vi "qrpostionM.vi"() -> ()   [LabVIEW 2019]
uses:
  <vilib>/vision/Instrument.llb/QR Code Report.ctl
  <vilib>/vision/Instrument.llb/QR Code Model Type.ctl
  <vilib>/vision/Instrument.llb/QR Code Stream Mode Type.ctl
  <vilib>/vision/Instrument.llb/Data Matrix Polarity.ctl
  <vilib>/vision/Instrument.llb/Demodulation Mode.ctl
  <vilib>/vision/Instrument.llb/Cell Sample Size.ctl
  <vilib>/vision/Instrument.llb/Cell Filter Mode.ctl
panel:
  out "Image Out 2":T1(plugin-control)
  in  "Stop (F)":bool
  out "Image Out":T1(plugin-control)
  out "Lx":dbl
  out "Rx":dbl
  out "Ly":i32
  out "Ry":i32
  out "QR Barcode Report (2D Barcode Reader 1)":T2={"Found?"=FALSE, "Data"="", "Bounding Box"=[], "Errors Corrected"=0, "Dimensions (Rows/Cols)"=0, "Version"=0, "QR Model"=3, "Stream Mode"=0, "Barcode Polarity"=-2, "Mirrored?"=FALSE, "Append Stream Position"=0, "Size of Append Stream"=0, "First EAN-128 ID"=0, "First Alternate Language ID"=0, "Append Stream ID"=0, "Minimum Edge Strength"=30, "Demodulation Mode"=-2, "Cell Sample Size"=-2, "Cell Filter Mode"=-2} {"Append Stream ID" format="%x"; "Cell Filter Mode" items=["Auto-detect"=-2, "Average"=0, "Median"=1, "Central Average"=2, "High Average"=3, "Low Average"=4, "Very High Average"=5, "Very Low Average"=6, "All Filters"=8]; "Cell Sample Size" items=["Auto-detect"=-2, "1x1"=1, "2x2"=2, "3x3"=3, "4x4"=4, "5x5"=5, "6x6"=6, "7x7"=7]; "Demodulation Mode" items=["Auto-detect"=-2, "Histogram"=0, "Local Contrast"=1, "Combination"=2, "All"=3]; "Barcode Polarity" items=["Auto-detect"=-2, "Black on White"=0, "White on Black"=1]; "Stream Mode" items=["Auto-detect", "Numeric", "AlphaNumeric", "Mixed", "Raw Bytes", "UCC/EAN-128 - In Tokens", "UCC/EAN-128 - In Data", "Extended Character Interpretation", "Kanji"]; "QR Model" items=["Auto Detect", "Micro", "Model 1", "Model 2"]; "Version" max=40 step=1}
  out "Data":string
  out "Array":string[][](array[string])
  out "Particle Measurements (Pixels) (Particle Analysis 1)":dbl[][](array[numeric]) format="%.2f"
  out "subarray":dbl[](array[numeric])
  out "min Y":dbl
  out "min X":dbl
  out "R1":string[](array[string])
  out "R2":string[](array[string])
  out "R3":string[](array[string])
  out "R4":string[](array[string])
  out "R5":string[](array[string])
  out "R11":string
  out "R12":string
  out "R21":string
  out "R22":string
  out "R31":string
  out "R32":string
  out "R41":string
  out "R42":string
  out "R51":string
  out "R52":string
  out "R13":string
  out "R14":string
  out "R15":string
  out "R23":string
  out "R24":string
  out "R25":string
  out "R33":string
  out "R34":string
  out "R35":string
  out "R43":string
  out "R44":string
  out "R45":string
  out "R53":string
  out "R54":string
  out "R55":string
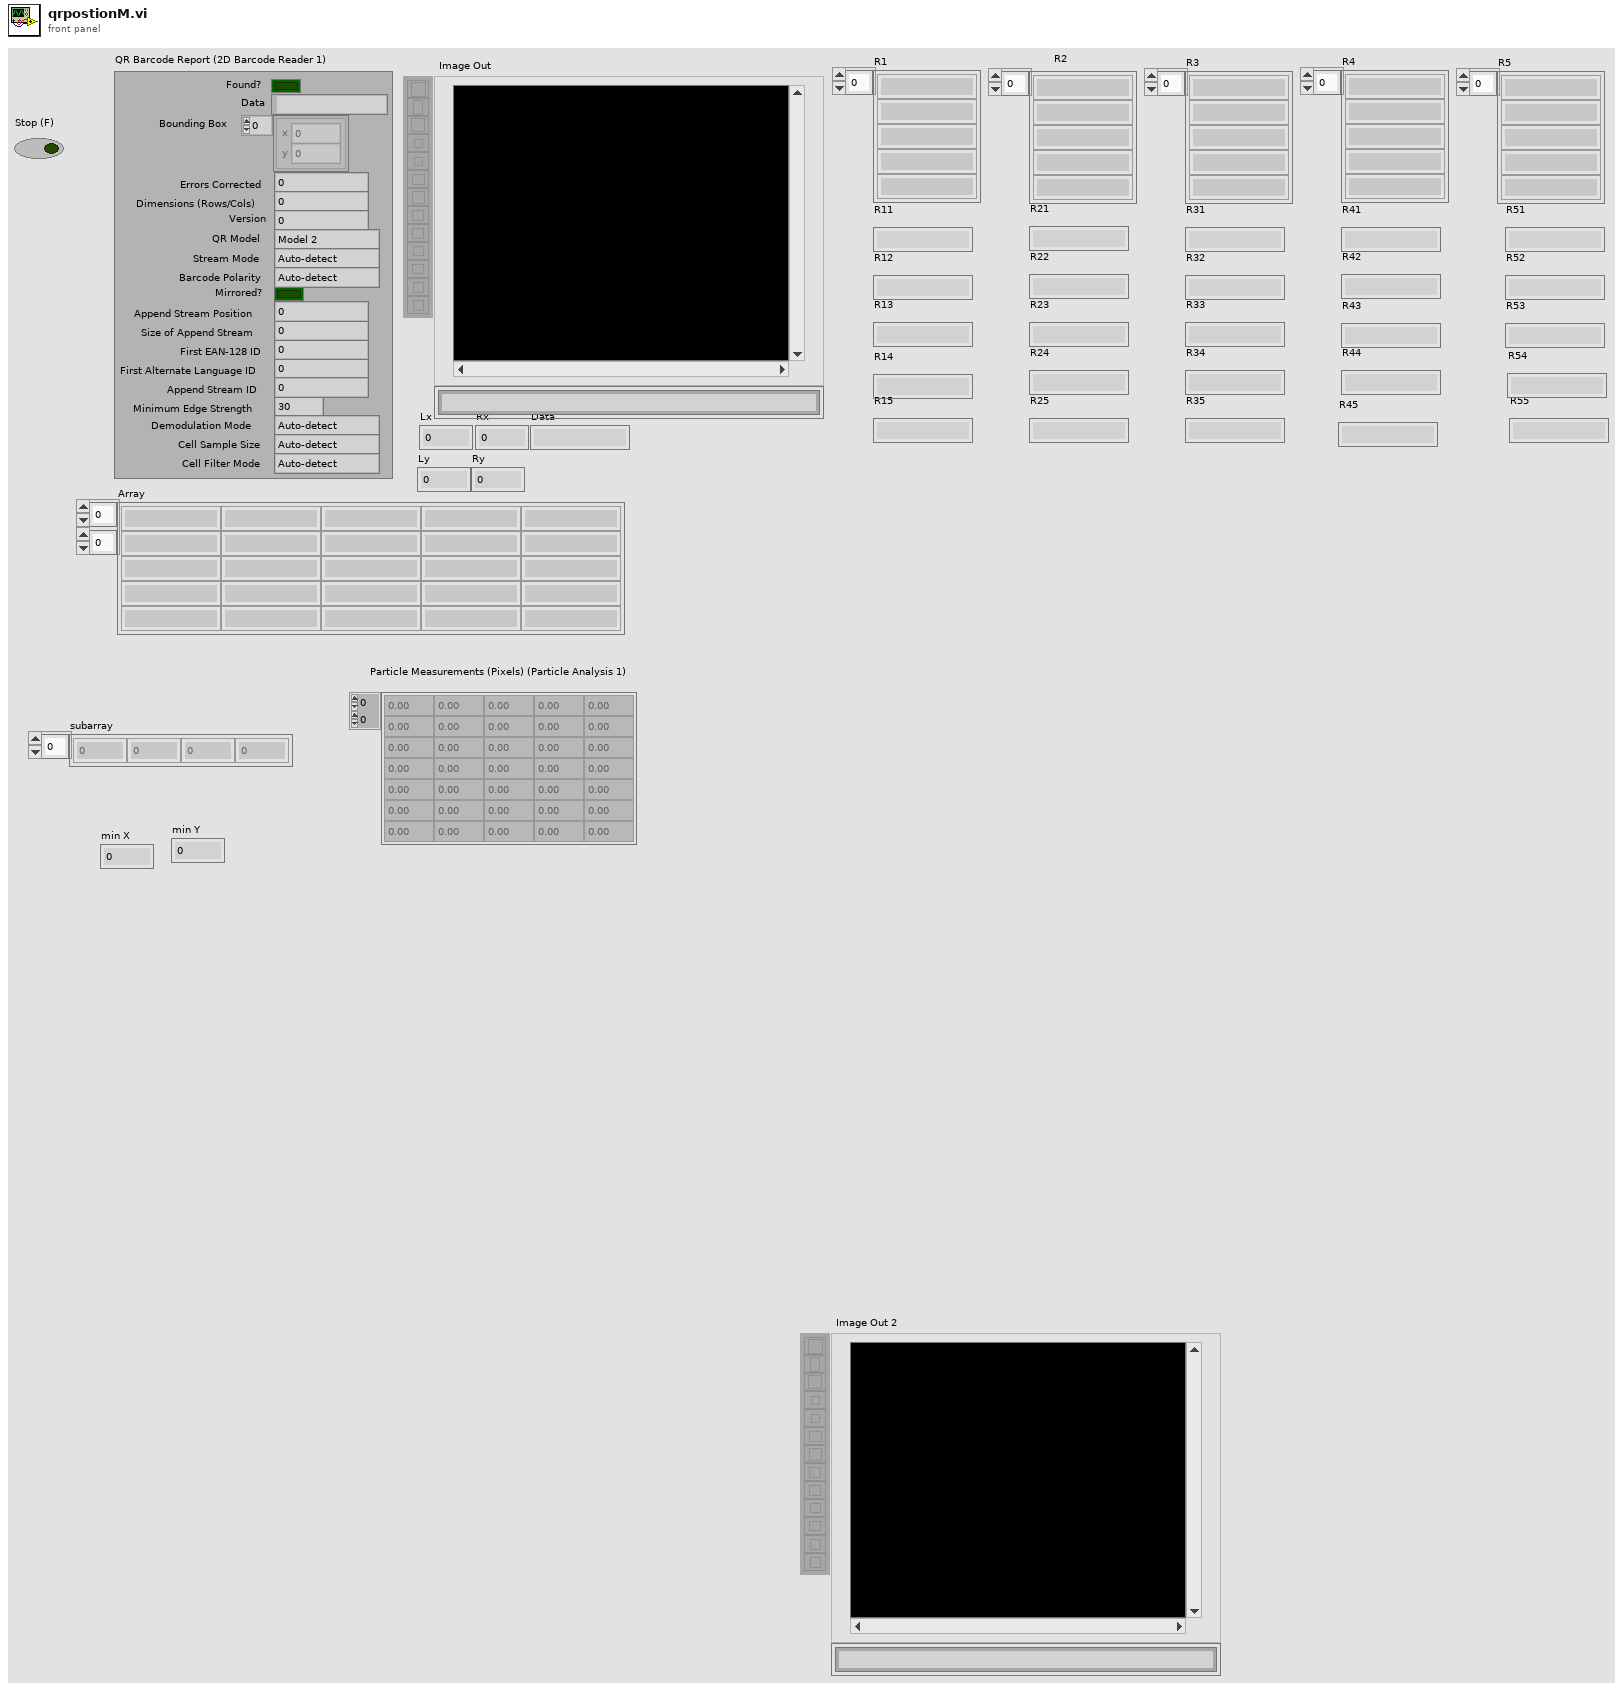
[diagram p1: front panel]
types:
  T1 = typedef "IMAQ Image.ctl" = refnum<image>
  T2 = typedef "QR Code Report.ctl" = cluster{"Found?":bool, "Data":string, "Bounding Box":cluster{"x":sgl, "y":sgl}[], "Errors Corrected":u32, "Dimensions (Rows/Cols)":u32, "Version":u32, "QR Model":T3, "Stream Mode":T4, "Barcode Polarity":T5, "Mirrored?":bool, "Append Stream Position":u32, "Size of Append Stream":u32, "First EAN-128 ID":i32, "First Alternate Language ID":i32, "Append Stream ID":u32, "Minimum Edge Strength":u32, "Demodulation Mode":T6, "Cell Sample Size":T7, "Cell Filter Mode":T8}
  T3 = typedef "QR Code Model Type.ctl" = i32
  T4 = typedef "QR Code Stream Mode Type.ctl" = i32
  T5 = typedef "Data Matrix Polarity.ctl" = i32
  T6 = typedef "Demodulation Mode.ctl" = i32
  T7 = typedef "Cell Sample Size.ctl" = i32
  T8 = typedef "Cell Filter Mode.ctl" = i32
  T9 = typedef "ROI Descriptor" = cluster{"Global Rectangle":i32[], "Contours":cluster{"ID":enum32{"External", "Internal"}, "Type":u32, "Coordinates":i32[]}[]}
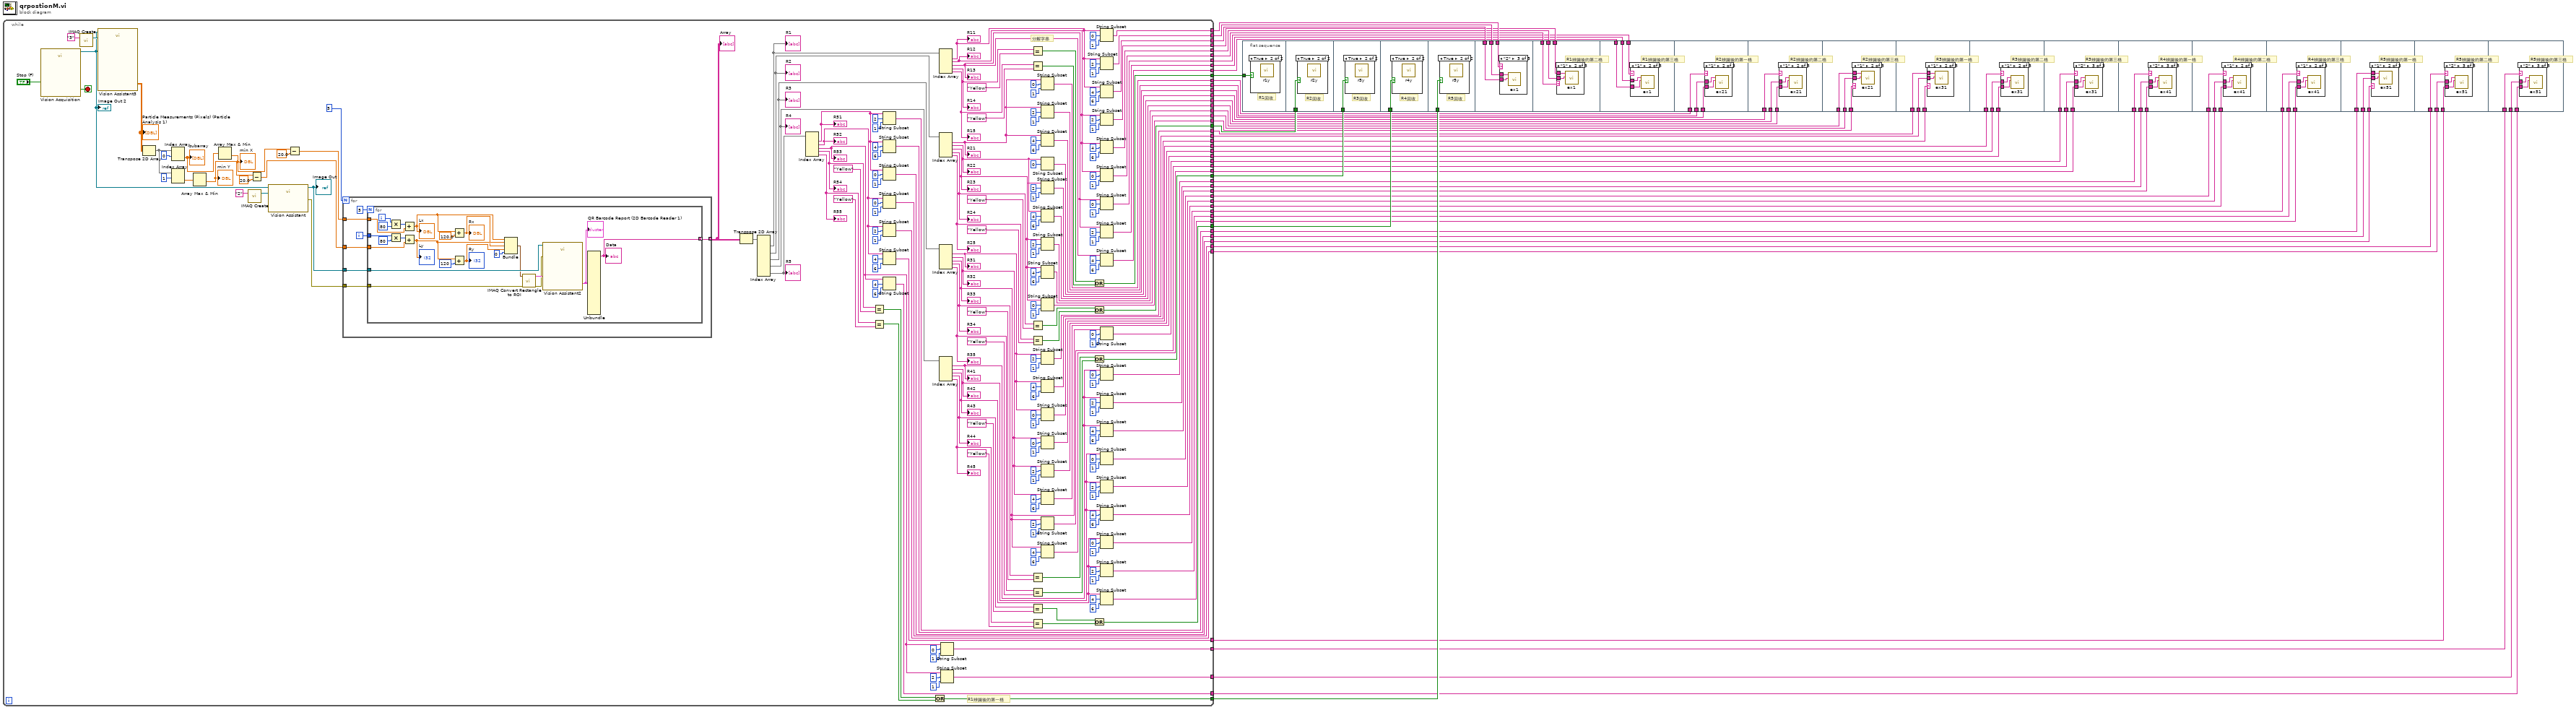
[diagram p0: block diagram]
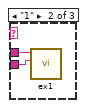
[diagram p8: hidden frame]
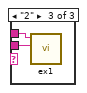
[diagram p10: hidden frame]
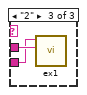
[diagram p12: hidden frame]
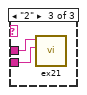
[diagram p14: hidden frame]
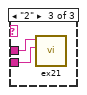
[diagram p16: hidden frame]
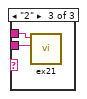
[diagram p18: hidden frame]
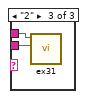
[diagram p20: hidden frame]
diagram:
  n1 = while {
    tunnel: [w100] -> w50
    tunnel: [w99] -> w49
    tunnel: [w98] -> w48
    tunnel: [w97] -> w47
    tunnel: [w96] -> w46
    tunnel: [w95] -> w45
    tunnel: [w94] -> w44
    tunnel: [w93] -> w43
    tunnel: [w92] -> w42
    tunnel: [w91] -> w41
    tunnel: [w90] -> w40
    tunnel: [w89] -> w39
    tunnel: [w88] -> w38
    tunnel: [w87] -> w37
    tunnel: [w86] -> w36
    tunnel: [w85] -> w35
    tunnel: [w84] -> w34
    tunnel: [w83] -> w33
    tunnel: [w82] -> w32
    tunnel: [w81] -> w31
    tunnel: [w80] -> w30
    tunnel: [w79] -> w29
    tunnel: [w78] -> w28
    tunnel: [w77] -> w27
    tunnel: [w76] -> w26
    tunnel: [w75] -> w25
    tunnel: [w74] -> w24
    tunnel: [w73] -> w23
    tunnel: [w72] -> w22
    tunnel: [w71] -> w21
    tunnel: [w70] -> w20
    tunnel: [w69] -> w19
    tunnel: [w68] -> w18
    tunnel: [w67] -> w17
    tunnel: [w66] -> w16
    tunnel: [w65] -> w15
    tunnel: [w64] -> w14
    tunnel: [w63] -> w13
    tunnel: [w62] -> w12
    tunnel: [w61] -> w11
    tunnel: [w60] -> w10
    tunnel: [w59] -> w9
    tunnel: [w58] -> w8
    tunnel: [w57] -> w7
    tunnel: [w56] -> w6
    tunnel: [w55] -> w5
    tunnel: [w54] -> w4
    tunnel: [w53] -> w3
    tunnel: [w52] -> w2
    tunnel: [w51] -> w1
    stop <- w262 stop-if-true
    # "R1辨識後的第一格"
    # "分解字串"
    n2 = call "Vision Acquisition"("Stop (F)"="Stop (F)") -> ("Image Out"=w240:T1, "Stopped"=w262:bool)  [unwired: 24 in, 1 out]
    "Image Out 2" <- w240
    n3 = call "IMAQ Create"("Image Name"="3") -> ("New Image"=w252:T1)  [unwired: 4 in, 1 out]
    n4 = call "Vision Assistant3"("Image In"=w240, "Image Dst"=w252) -> ("Particle Measurements (Pixels) (Particle Analysis 1)"=w253:dbl[][])  [unwired: 22 in, 3 out]
    "Particle Measurements (Pixels) (Particle Analysis 1)" <- w253
    n5 = Transpose 2D Array(2D array=w253) -> (transposed array=w254:dbl[][])
    n6 = Index Array(array=w254, index (row)=0) -> (element=w256:dbl[])  [unwired: 1 in]
    "subarray" <- w256
    n7 = Index Array(array=w254, index (row)=1) -> (element=w255:dbl[])  [unwired: 1 in]
    n8 = Array Max & Min(array=w255) -> (min value=w258:dbl)  [unwired: 3 out]
    "min Y" <- w258
    n9 = Array Max & Min(array=w256) -> (min value=w257:dbl)  [unwired: 3 out]
    "min X" <- w257
    n10 = call "IMAQ Create"("Image Name"="2") -> ("New Image"=w250:T1)  [unwired: 4 in, 1 out]
    n11 = Subtract(x=w258, y=20.0) -> (x-y=w259:dbl)
    n12 = call "Vision Assistant"("Image In"=w240, "Image Dst"=w250) -> ("Image Out"=w251:T1, "error out"=w249:errorcluster)  [unwired: 24 in]
    "Image Out" <- w251
    n13 = Subtract(x=w257, y=20.0) -> (x-y=w248:dbl)
    n14 = for {
      N: 5 -> [_]
      tunnel: w251 -> [w269]
      tunnel: w248 -> [w267]
      tunnel: w249 -> [w266]
      tunnel: [w265] -> w260 mode=indexing
      tunnel: w259 -> [w264]
      i -> [w268]
      n15 = for {
        N: 5 -> [_]
        tunnel: w269 -> [w292]
        tunnel: w268 -> [w272]
        tunnel: w267 -> [w288]
        tunnel: w266 -> [w276]
        tunnel: [w274] -> w265 mode=indexing
        tunnel: w264 -> [w271]
        i -> [w273]
        n16 = Multiply(x=w273, y=80) -> (x*y=w289:i32)
        n17 = Multiply(x=w272, y=80) -> (x*y=w286:i32)
        n18 = Add(x=w289, y=w288) -> (x+y=w283:dbl)
        "Lx" <- w283
        n19 = Add(x=w286, y=w271) -> (x+y=w282:dbl)
        "Ly" <- w282
        n20 = Add(x=w283, y=120.0) -> (x+y=w281:dbl)
        "Rx" <- w281
        n21 = Add(x=w282, y=120) -> (x+y=w280:dbl)
        "Ry" <- w280
        n22 = Bundle(w283, w282, w281, w280, 0) -> (w278:cluster{dbl, dbl, dbl, dbl, i32})  [unwired: 1 in]
        n23 = call "IMAQ Convert Rectangle to ROI"("error in (no error)"=w276, "Rectangle"=w278) -> ("error out"=w277:errorcluster, "ROI Descriptor"=w291:T9)  [unwired: 7 in]
        n24 = call "Vision Assistant2"("Image In"=w292, "ROI Descriptor (2D Barcode Reader 1)"=w291, "error in"=w277) -> ("QR Barcode Report (2D Barcode Reader 1)"=w275:T2)  [unwired: 22 in, 2 out]
        "QR Barcode Report (2D Barcode Reader 1)" <- w275
        n25 = Unbundle(w275) -> ("Data"=w274:string)  [unwired: 18 out]
        "Data" <- w274
      }
    }
    "Array" <- w260
    n26 = Transpose 2D Array(2D array=w260) -> (transposed array=w261:string[][])
    n27 = Index Array(array=w261) -> (element #1=w235:string[], element #2=w239:string[], element #3=w237:string[], element #4=w236:string[], element #5=w238:string[])  [unwired: 10 in]
    "R1" <- w235
    "R2" <- w239
    "R3" <- w237
    "R4" <- w236
    "R5" <- w238
    n28 = Index Array(array=w238) -> (element #1=w119:string, element #2=w112:string, element #3=w105:string, element #4=w205:string, element #5=w206:string)  [unwired: 5 in]
    "R51" <- w119
    "R52" <- w112
    "R53" <- w105
    "R54" <- w205
    "R55" <- w206
    n29 = Equal?(x=w205, y="Yellow") -> (x = y?=w209:bool)
    n30 = Equal?(x=w206, y="Yellow") -> (x = y?=w208:bool)
    n31 = String Subset(string=w119, offset (0)=2, length (rest)=1 ("length (rest)")) -> (substring=w58:string)
    n32 = String Subset(string=w119, offset (0)=4, length (rest)=6 ("length (rest)")) -> (substring=w57:string)
    n33 = String Subset(string=w119, offset (0)=0, length (rest)=1 ("length (rest)")) -> (substring=w59:string)
    n34 = String Subset(string=w112, offset (0)=0, length (rest)=1 ("length (rest)")) -> (substring=w56:string)
    n35 = String Subset(string=w112, offset (0)=2, length (rest)=1 ("length (rest)")) -> (substring=w55:string)
    n36 = String Subset(string=w112, offset (0)=4, length (rest)=6 ("length (rest)")) -> (substring=w54:string)
    n37 = String Subset(string=w105, offset (0)=4, length (rest)=6 ("length (rest)")) -> (substring=w51:string)
    n38 = Or(x=w209, y=w208) -> (x .or. y?=w96:bool)
    n39 = Index Array(array=w239) -> (element #1=w181:string, element #2=w175:string, element #3=w169:string, element #4=w224:string, element #5=w223:string)  [unwired: 5 in]
    "R21" <- w181
    "R22" <- w175
    "R23" <- w169
    "R24" <- w224
    "R25" <- w223
    n40 = Index Array(array=w237) -> (element #1=w161:string, element #2=w154:string, element #3=w147:string, element #4=w217:string, element #5=w218:string)  [unwired: 5 in]
    "R31" <- w161
    "R32" <- w154
    "R33" <- w147
    "R34" <- w217
    "R35" <- w218
    n41 = Index Array(array=w236) -> (element #1=w140:string, element #2=w133:string, element #3=w126:string, element #4=w213:string, element #5=w211:string)  [unwired: 5 in]
    "R41" <- w140
    "R42" <- w133
    "R43" <- w126
    "R44" <- w213
    "R45" <- w211
    n42 = Index Array(array=w235) -> (element #1=w202:string, element #2=w195:string, element #3=w188:string, element #4=w234:string, element #5=w232:string)  [unwired: 5 in]
    "R11" <- w202
    "R12" <- w195
    "R13" <- w188
    "R14" <- w234
    "R15" <- w232
    n43 = String Subset(string=w105, offset (0)=0, length (rest)=1 ("length (rest)")) -> (substring=w53:string)
    n44 = String Subset(string=w105, offset (0)=2, length (rest)=1 ("length (rest)")) -> (substring=w52:string)
    n45 = Equal?(x=w234, y="Yellow") -> (x = y?=w230:bool)
    n46 = Equal?(x=w232, y="Yellow") -> (x = y?=w229:bool)
    n47 = Equal?(x=w224, y="Yellow") -> (x = y?=w227:bool)
    n48 = Equal?(x=w223, y="Yellow") -> (x = y?=w226:bool)
    n49 = Equal?(x=w217, y="Yellow") -> (x = y?=w221:bool)
    n50 = Equal?(x=w218, y="Yellow") -> (x = y?=w220:bool)
    n51 = Equal?(x=w213, y="Yellow") -> (x = y?=w215:bool)
    n52 = Equal?(x=w211, y="Yellow") -> (x = y?=w214:bool)
    n53 = String Subset(string=w181, offset (0)=0, length (rest)=1 ("length (rest)")) -> (substring=w86:string)
    n54 = String Subset(string=w181, offset (0)=2, length (rest)=1 ("length (rest)")) -> (substring=w85:string)
    n55 = String Subset(string=w181, offset (0)=4, length (rest)=6 ("length (rest)")) -> (substring=w84:string)
    n56 = String Subset(string=w175, offset (0)=0) -> (substring=w83:string)  [unwired: 1 in]
    n57 = String Subset(string=w175, offset (0)=2, length (rest)=1 ("length (rest)")) -> (substring=w82:string)
    n58 = String Subset(string=w175, offset (0)=4, length (rest)=6 ("length (rest)")) -> (substring=w81:string)
    n59 = String Subset(string=w169, offset (0)=2, length (rest)=1 ("length (rest)")) -> (substring=w79:string)
    n60 = String Subset(string=w169, offset (0)=4, length (rest)=6 ("length (rest)")) -> (substring=w78:string)
    n61 = String Subset(string=w169, offset (0)=0, length (rest)=1 ("length (rest)")) -> (substring=w80:string)
    n62 = String Subset(string=w161, offset (0)=2, length (rest)=1 ("length (rest)")) -> (substring=w76:string)
    n63 = String Subset(string=w161, offset (0)=4, length (rest)=6 ("length (rest)")) -> (substring=w75:string)
    n64 = String Subset(string=w161, offset (0)=0, length (rest)=1 ("length (rest)")) -> (substring=w77:string)
    n65 = String Subset(string=w154, offset (0)=0, length (rest)=1 ("length (rest)")) -> (substring=w74:string)
    n66 = String Subset(string=w154, offset (0)=2, length (rest)=1 ("length (rest)")) -> (substring=w73:string)
    n67 = String Subset(string=w154, offset (0)=4, length (rest)=6 ("length (rest)")) -> (substring=w72:string)
    n68 = String Subset(string=w147, offset (0)=2, length (rest)=1 ("length (rest)")) -> (substring=w70:string)
    n69 = String Subset(string=w147, offset (0)=4, length (rest)=6 ("length (rest)")) -> (substring=w69:string)
    n70 = Or(x=w230, y=w229) -> (x .or. y?=w100:bool)
    n71 = Or(x=w227, y=w226) -> (x .or. y?=w99:bool)
    n72 = Or(x=w221, y=w220) -> (x .or. y?=w98:bool)
    n73 = Or(x=w215, y=w214) -> (x .or. y?=w97:bool)
    n74 = String Subset(string=w202, offset (0)=0, length (rest)=1 ("length (rest)")) -> (substring=w95:string)
    n75 = String Subset(string=w202, offset (0)=2, length (rest)=1 ("length (rest)")) -> (substring=w94:string)
    n76 = String Subset(string=w202, offset (0)=4, length (rest)=6 ("length (rest)")) -> (substring=w93:string)
    n77 = String Subset(string=w195, offset (0)=2, length (rest)=1 ("length (rest)")) -> (substring=w91:string)
    n78 = String Subset(string=w195, offset (0)=4, length (rest)=6 ("length (rest)")) -> (substring=w90:string)
    n79 = String Subset(string=w195, offset (0)=0, length (rest)=1 ("length (rest)")) -> (substring=w92:string)
    n80 = String Subset(string=w188, offset (0)=0, length (rest)=1 ("length (rest)")) -> (substring=w89:string)
    n81 = String Subset(string=w188, offset (0)=2, length (rest)=1 ("length (rest)")) -> (substring=w88:string)
    n82 = String Subset(string=w188, offset (0)=4, length (rest)=6 ("length (rest)")) -> (substring=w87:string)
    n83 = String Subset(string=w147, offset (0)=0, length (rest)=1 ("length (rest)")) -> (substring=w71:string)
    n84 = String Subset(string=w140, offset (0)=0, length (rest)=1 ("length (rest)")) -> (substring=w68:string)
    n85 = String Subset(string=w140, offset (0)=2, length (rest)=1 ("length (rest)")) -> (substring=w67:string)
    n86 = String Subset(string=w140, offset (0)=4, length (rest)=6 ("length (rest)")) -> (substring=w66:string)
    n87 = String Subset(string=w133, offset (0)=0, length (rest)=1 ("length (rest)")) -> (substring=w65:string)
    n88 = String Subset(string=w133, offset (0)=2, length (rest)=1 ("length (rest)")) -> (substring=w64:string)
    n89 = String Subset(string=w133, offset (0)=4, length (rest)=6 ("length (rest)")) -> (substring=w63:string)
    n90 = String Subset(string=w126, offset (0)=0, length (rest)=1 ("length (rest)")) -> (substring=w62:string)
    n91 = String Subset(string=w126, offset (0)=2, length (rest)=1 ("length (rest)")) -> (substring=w61:string)
    n92 = String Subset(string=w126, offset (0)=4, length (rest)=6 ("length (rest)")) -> (substring=w60:string)
  }
  n93 = flat-sequence {
    tunnel: w50 -> [w293]
    tunnel: w49 -> [w294]
    tunnel: w48 -> [w295]
    tunnel: w47 -> [w296]
    tunnel: w46 -> [w297]
    tunnel: w45 -> [w300]
    tunnel: w44 -> [w299]
    tunnel: w43 -> [w298]
    tunnel: w42 -> [w307]
    tunnel: w41 -> [w306]
    tunnel: w40 -> [w305]
    tunnel: w39 -> [w314]
    tunnel: w38 -> [w313]
    tunnel: w37 -> [w312]
    tunnel: w36 -> [w321]
    tunnel: w35 -> [w320]
    tunnel: w34 -> [w319]
    tunnel: w33 -> [w328]
    tunnel: w32 -> [w327]
    tunnel: w31 -> [w326]
    tunnel: w30 -> [w335]
    tunnel: w29 -> [w334]
    tunnel: w28 -> [w333]
    tunnel: w27 -> [w342]
    tunnel: w26 -> [w341]
    tunnel: w25 -> [w340]
    tunnel: w24 -> [w349]
    tunnel: w23 -> [w348]
    tunnel: w22 -> [w347]
    tunnel: w21 -> [w356]
    tunnel: w20 -> [w355]
    tunnel: w19 -> [w354]
    tunnel: w18 -> [w361]
    tunnel: w17 -> [w362]
    tunnel: w16 -> [w363]
    tunnel: w15 -> [w370]
    tunnel: w14 -> [w369]
    tunnel: w13 -> [w368]
    tunnel: w12 -> [w377]
    tunnel: w11 -> [w376]
    tunnel: w10 -> [w375]
    tunnel: w9 -> [w384]
    tunnel: w8 -> [w383]
    tunnel: w7 -> [w382]
    tunnel: w6 -> [w391]
    tunnel: w5 -> [w390]
    tunnel: w4 -> [w389]
    tunnel: w3 -> [w398]
    tunnel: w2 -> [w397]
    tunnel: w1 -> [w396]
    frame #0 {
      # "R1回收"
      n94 = case shown="True" w293 {
        frame False {
        }
        frame True {
          n95 = call "r1y.vi"() -> ()  [unwired: 12 in]
        }
      }
    }
    frame #1 {
      # "R2回收"
      n96 = case shown="True" w294 {
        frame False {
        }
        frame True {
          n97 = call "r2y.vi"() -> ()  [unwired: 12 in]
        }
      }
    }
    frame #2 {
      # "R3回收"
      n98 = case shown="True" w295 {
        frame False {
        }
        frame True {
          n99 = call "r3y.vi"() -> ()  [unwired: 12 in]
        }
      }
    }
    frame #3 {
      # "R4回收"
      n100 = case shown="True" w296 {
        frame False {
        }
        frame True {
          n101 = call "r4y.vi"() -> ()  [unwired: 12 in]
        }
      }
    }
    frame #4 {
      # "R5回收"
      n102 = case shown="True" w297 {
        frame False {
        }
        frame True {
          n103 = call "r5y.vi"() -> ()  [unwired: 12 in]
        }
      }
    }
    frame #5 {
      n104 = case shown="\"2\"" w300 {
        tunnel: w299 -> [_ w301 w304]
        tunnel: w298 -> [_ w302 w303]
        frame "0", Default {
        }
        frame "1" {
          n105 = call "ex1.vi"("Data"=w302, "Data 2"=w301) -> ()  [unwired: 10 in]
        }
        frame "2" {
          n106 = call "ex1.vi"("Data"=w303, "Data 2"=w304) -> ()  [unwired: 10 in]
        }
      }
    }
    frame #6 {
      # "R1辨識後的第二格"
      n107 = case shown="\"1\"" w307 {
        tunnel: w306 -> [_ w308 w311]
        tunnel: w305 -> [_ w309 w310]
        frame "0", Default {
        }
        frame "1" {
          n108 = call "ex1.vi"("Data"=w309, "Data 2"=w308) -> ()  [unwired: 10 in]
        }
        frame "2" {
          n109 = call "ex1.vi"("Data"=w310, "Data 2"=w311) -> ()  [unwired: 10 in]
        }
      }
    }
    frame #7 {
      # "R1辨識後的第三格"
      n110 = case shown="\"1\"" w314 {
        tunnel: w313 -> [_ w315 w318]
        tunnel: w312 -> [_ w316 w317]
        frame "0", Default {
        }
        frame "1" {
          n111 = call "ex1.vi"("Data"=w316, "Data 2"=w315) -> ()  [unwired: 10 in]
        }
        frame "2" {
          n112 = call "ex1.vi"("Data"=w318, "Data 2"=w317) -> ()  [unwired: 10 in]
        }
      }
    }
    frame #8 {
      # "R2辨識後的第一格"
      n113 = case shown="\"1\"" w321 {
        tunnel: w320 -> [_ w322 w325]
        tunnel: w319 -> [_ w323 w324]
        frame "0", Default {
        }
        frame "1" {
          n114 = call "ex21.vi"("Data"=w323, "Data 2"=w322) -> ()  [unwired: 10 in]
        }
        frame "2" {
          n115 = call "ex21.vi"("Data"=w324, "Data 2"=w325) -> ()  [unwired: 10 in]
        }
      }
    }
    frame #9 {
      # "R2辨識後的第二格"
      n116 = case shown="\"1\"" w328 {
        tunnel: w327 -> [_ w329 w331]
        tunnel: w326 -> [_ w330 w332]
        frame "0", Default {
        }
        frame "1" {
          n117 = call "ex21.vi"("Data"=w330, "Data 2"=w329) -> ()  [unwired: 10 in]
        }
        frame "2" {
          n118 = call "ex21.vi"("Data"=w332, "Data 2"=w331) -> ()  [unwired: 10 in]
        }
      }
    }
    frame #10 {
      # "R2辨識後的第三格"
      n119 = case shown="\"1\"" w335 {
        tunnel: w334 -> [_ w336 w338]
        tunnel: w333 -> [_ w337 w339]
        frame "0", Default {
        }
        frame "1" {
          n120 = call "ex21.vi"("Data"=w337, "Data 2"=w336) -> ()  [unwired: 10 in]
        }
        frame "2" {
          n121 = call "ex21.vi"("Data"=w339, "Data 2"=w338) -> ()  [unwired: 10 in]
        }
      }
    }
    frame #11 {
      # "R3辨識後的第一格"
      n122 = case shown="\"1\"" w342 {
        tunnel: w341 -> [_ w343 w346]
        tunnel: w340 -> [_ w344 w345]
        frame "0", Default {
        }
        frame "1" {
          n123 = call "ex31.vi"("Data"=w344, "Data 2"=w343) -> ()  [unwired: 10 in]
        }
        frame "2" {
          n124 = call "ex31.vi"("Data"=w345, "Data 2"=w346) -> ()  [unwired: 10 in]
        }
      }
    }
    frame #12 {
      # "R3辨識後的第二格"
      n125 = case shown="\"1\"" w349 {
        tunnel: w348 -> [_ w350 w352]
        tunnel: w347 -> [_ w351 w353]
        frame "0", Default {
        }
        frame "1" {
          n126 = call "ex31.vi"("Data"=w351, "Data 2"=w350) -> ()  [unwired: 10 in]
        }
        frame "2" {
          n127 = call "ex31.vi"("Data"=w353, "Data 2"=w352) -> ()  [unwired: 10 in]
        }
      }
    }
    frame #13 {
      # "R3辨識後的第三格"
      n128 = case shown="\"2\"" w356 {
        tunnel: w355 -> [_ w357 w359]
        tunnel: w354 -> [_ w358 w360]
        frame "0", Default {
        }
        frame "1" {
          n129 = call "ex31.vi"("Data"=w358, "Data 2"=w357) -> ()  [unwired: 10 in]
        }
        frame "2" {
          n130 = call "ex31.vi"("Data"=w360, "Data 2"=w359) -> ()  [unwired: 10 in]
        }
      }
    }
    frame #14 {
      # "R4辨識後的第一格"
      n131 = case shown="\"2\"" w361 {
        tunnel: w363 -> [_ w364 w366]
        tunnel: w362 -> [_ w365 w367]
        frame "0", Default {
        }
        frame "1" {
          n132 = call "ex41.vi"("Data"=w364, "Data 2"=w365) -> ()  [unwired: 10 in]
        }
        frame "2" {
          n133 = call "ex41.vi"("Data"=w366, "Data 2"=w367) -> ()  [unwired: 10 in]
        }
      }
    }
    frame #15 {
      # "R4辨識後的第二格"
      n134 = case shown="\"1\"" w370 {
        tunnel: w369 -> [_ w372 w374]
        tunnel: w368 -> [_ w371 w373]
        frame "0", Default {
        }
        frame "1" {
          n135 = call "ex41.vi"("Data"=w371, "Data 2"=w372) -> ()  [unwired: 10 in]
        }
        frame "2" {
          n136 = call "ex41.vi"("Data"=w373, "Data 2"=w374) -> ()  [unwired: 10 in]
        }
      }
    }
    frame #16 {
      # "R4辨識後的第三格"
      n137 = case shown="\"1\"" w377 {
        tunnel: w376 -> [_ w379 w381]
        tunnel: w375 -> [_ w378 w380]
        frame "0", Default {
        }
        frame "1" {
          n138 = call "ex41.vi"("Data"=w378, "Data 2"=w379) -> ()  [unwired: 10 in]
        }
        frame "2" {
          n139 = call "ex41.vi"("Data"=w380, "Data 2"=w381) -> ()  [unwired: 10 in]
        }
      }
    }
    frame #17 {
      # "R5辨識後的第一格"
      n140 = case shown="\"1\"" w384 {
        tunnel: w383 -> [_ w385 w388]
        tunnel: w382 -> [_ w386 w387]
        frame "0", Default {
        }
        frame "1" {
          n141 = call "ex51.vi"("Data"=w386, "Data 2"=w385) -> ()  [unwired: 10 in]
        }
        frame "2" {
          n142 = call "ex51.vi"("Data"=w387, "Data 2"=w388) -> ()  [unwired: 10 in]
        }
      }
    }
    frame #18 {
      # "R5辨識後的第二格"
      n143 = case shown="\"2\"" w391 {
        tunnel: w390 -> [_ w392 w394]
        tunnel: w389 -> [_ w393 w395]
        frame "0", Default {
        }
        frame "1" {
          n144 = call "ex51.vi"("Data"=w393, "Data 2"=w392) -> ()  [unwired: 10 in]
        }
        frame "2" {
          n145 = call "ex51.vi"("Data"=w395, "Data 2"=w394) -> ()  [unwired: 10 in]
        }
      }
    }
    frame #19 {
      # "R5辨識後的第三格"
      n146 = case shown="\"2\"" w398 {
        tunnel: w397 -> [_ w399 w401]
        tunnel: w396 -> [_ w400 w402]
        frame "0", Default {
        }
        frame "1" {
          n147 = call "ex51.vi"("Data"=w400, "Data 2"=w399) -> ()  [unwired: 10 in]
        }
        frame "2" {
          n148 = call "ex51.vi"("Data"=w402, "Data 2"=w401) -> ()  [unwired: 10 in]
        }
      }
    }
  }
